vi "Paul_trap_scan.vi"() -> ()   [LabVIEW 2018]
uses:
  <instrlib>/AFG-2225/AFG-2225.lvlib
panel:
  in  "base name":string
  in  "Directory path":path=path "F:/data/20220803/3um_SiO2/1/pump/1"
  in  "stop 2 channels":bool
  in  "Single channel":bool
  in  "stop":bool
  in  "number of tests, Frequency":dbl
  in  "number of tests, Voltage":dbl
  in  "Frequency Step(kHz)":dbl=3.0 format="%.3g"
  in  "Voltage Step(V)":dbl=3.0 format="%.3g"
  in  "Delay Time 4+ (s)":dbl=1.0 caption="Delay Time (s)"
  in  "DC Offset (0.00 V)":dbl format="%.2g"
  in  "Frequency (kHz)":dbl=1000.0 format="%_7g"
  in  "Start Voltage (Vpp)":dbl=3.0 format="%.3g"
  in  "Waveform Function (0: Sine)":u16(ring) items=["Sine", "Square", "Pulse", "Ramp", "Noise"]
  in  "Impedance (0: 50 OHM)":u16(ring) items=["50 OHM", "High Z"]
  in  "Channel (0: CH1)":u16(ring) items=["CH1", "CH2"]
  # "Wait for a loop to end then stop"
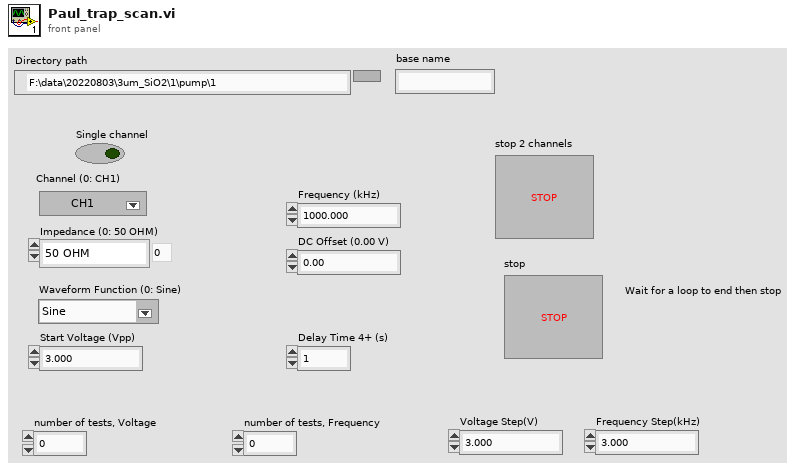
[diagram p1: front panel]
types:
  T1 = enum16{"open", "replace", "create", "open or create", "replace or create", "replace or create with confirmation"}
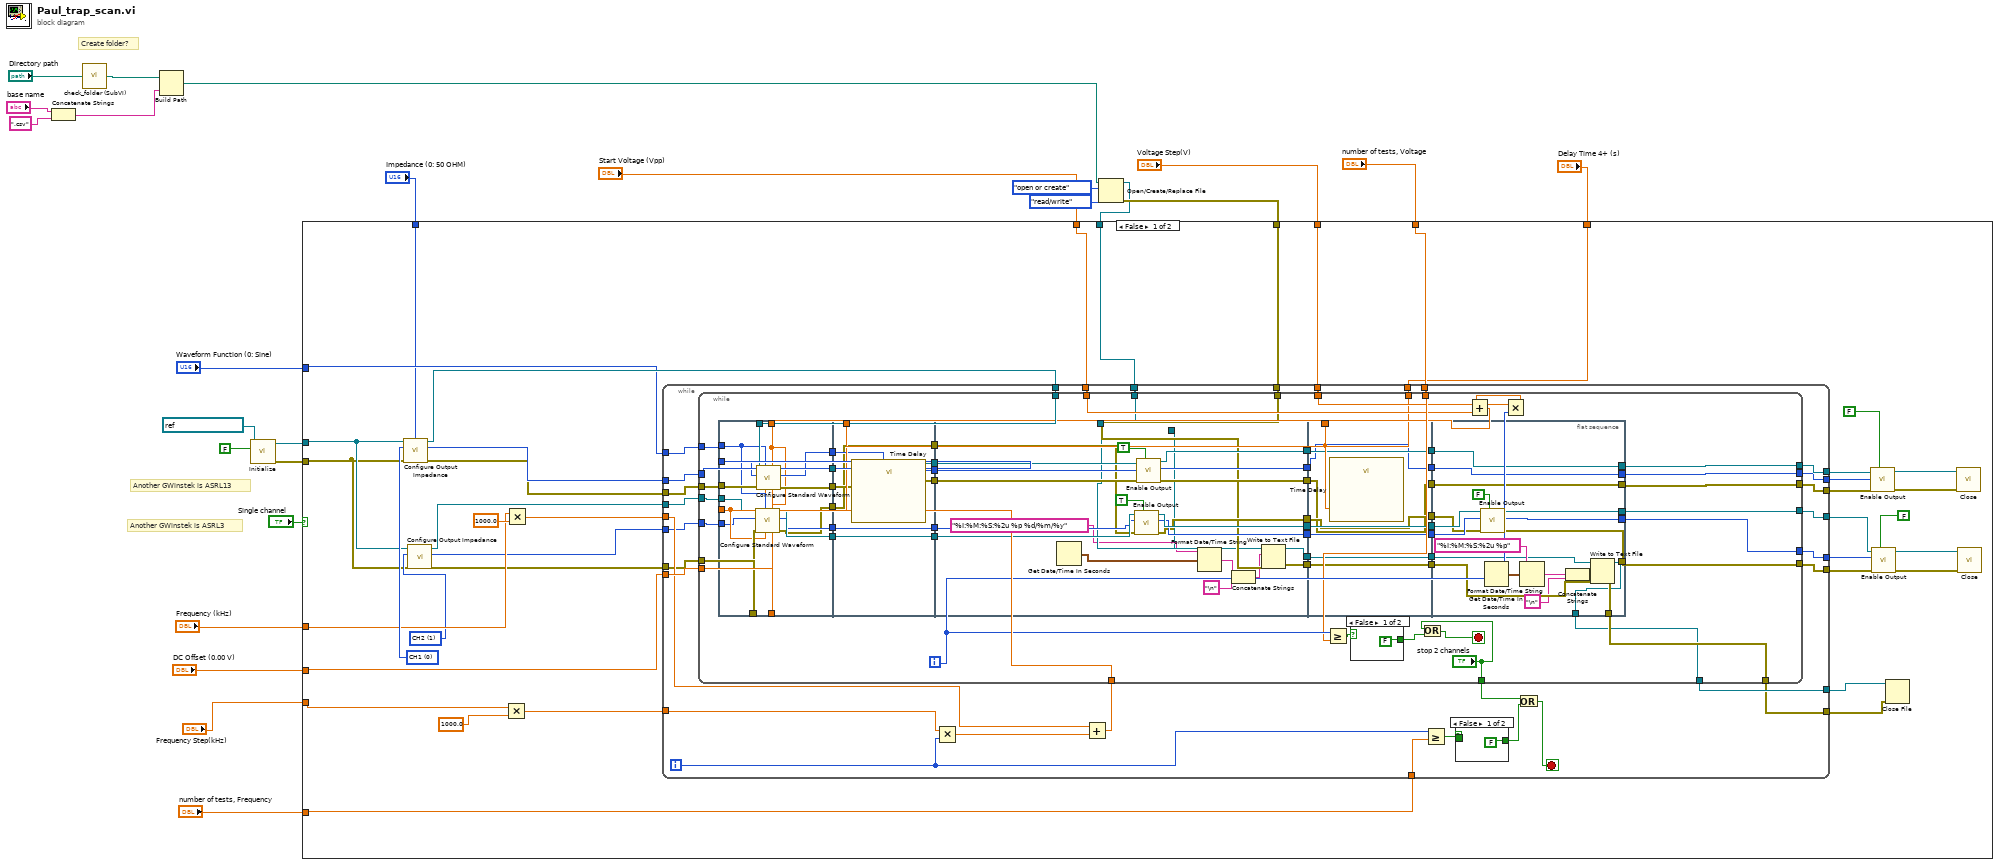
[diagram p0: block diagram]
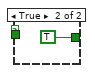
[diagram p2: hidden frame]
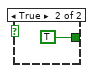
[diagram p3: hidden frame]
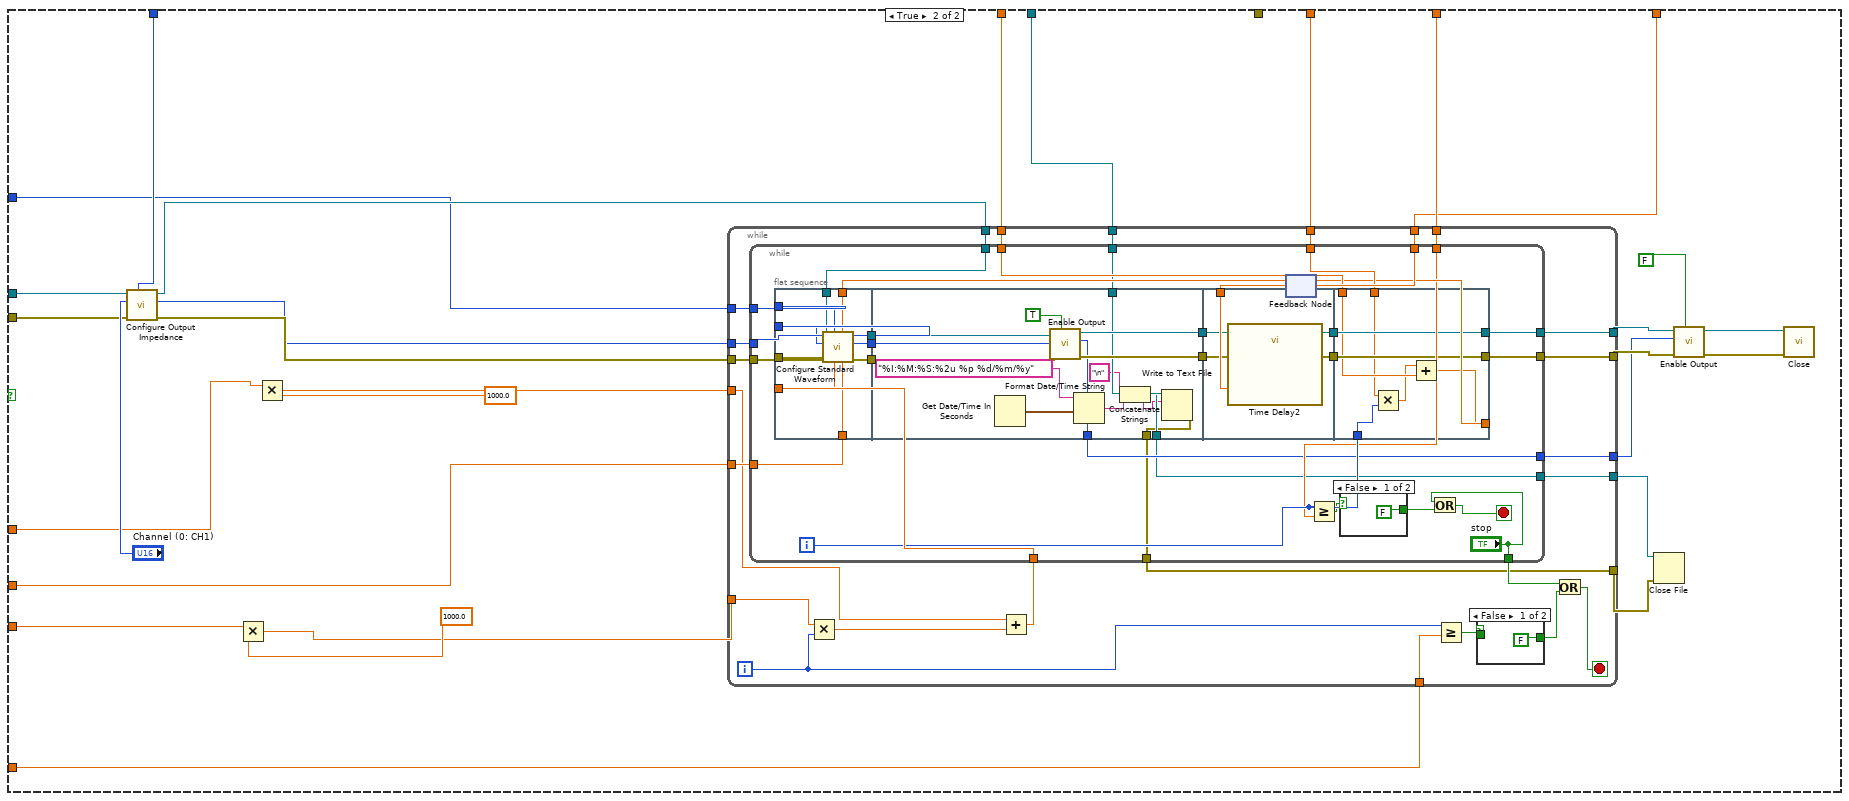
[diagram p4: hidden frame]
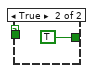
[diagram p5: hidden frame]
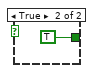
[diagram p6: hidden frame]
diagram:
  # "Create folder?"
  # "Another GWinstek is ASRL3"
  # "Another GWinstek is ASRL13"
  n1 = Concatenate Strings("base name", ".csv" ("string")) -> (w8:string)
  n2 = call "check_folder (SubVI).vi"("path in"="Directory path") -> ("path out"=w6:path)
  n3 = Build Path(base path=w6, name or relative path=w8) -> (appended path=w4:path)
  n4 = call <instrlib>:"Initialize.vi"("ID Query (True)"=FALSE, "VISA resource name"=refnum<visa-resource-name> "ASRL13::INSTR") -> ("error out"=w23:errorcluster, "VISA resource name out"=w24:refnum<visa-resource-name>)  [unwired: 8 in]
  n5 = Open/Create/Replace File(file path (use dialog)=w4, operation (0:open)=T1."open or create", access (0:read/write)=enum16{"read/write", "read-only", "write-only"}."read/write") -> (refnum out=w3:refnum<file>, error out=w5:errorcluster)  [unwired: 3 in, 1 out]
  n6 = case shown="False" "Single channel" {
    tunnel: w24 -> [w42 w261]
    tunnel: w23 -> [w41 w260]
    tunnel: "Impedance (0: 50 OHM)" -> [w30 w246]
    tunnel: "Start Voltage (Vpp)" -> [w52 w245]
    tunnel: "Voltage Step(V)" -> [w51 w244]
    tunnel: "number of tests, Voltage" -> [w50 w243]
    tunnel: "Delay Time 4+ (s)" -> [w49 w242]
    tunnel: "Waveform Function (0: Sine)" -> [w44 w241]
    tunnel: "Frequency (kHz)" -> [w45 w240]
    tunnel: "DC Offset (0.00 V)" -> [w46 w239]
    tunnel: "Frequency Step(kHz)" -> [w47 w238]
    tunnel: "number of tests, Frequency" -> [w48 w237]
    tunnel: w3 -> [w29 w236]
    tunnel: w5 -> [w28 _]
    frame False {
      w56 = u16 0 items=["CH1", "CH2"] ("Channel (0: CH1)")
      w43 = u16 1 items=["CH1", "CH2"] ("Channel (0: CH1)")
      n7 = call <instrlib>:"Configure Output Impedance.vi"("VISA resource name"=w42, "Channel (0: CH1)"=w56, "error in (no error)"=w41, "Impedance (0: 50 OHM)"=w30) -> ("VISA resource name out"=w59:refnum<visa-resource-name>, "Channel out"=w58:u16, "error out"=w57:errorcluster)  [unwired: 4 in]
      n8 = call <instrlib>:"Configure Output Impedance.vi"("VISA resource name"=w42, "Channel (0: CH1)"=w43, "error in (no error)"=w41) -> ("VISA resource name out"=w40:refnum<visa-resource-name>, "Channel out"=w31:u16, "error out"=w39:errorcluster)  [unwired: 5 in]
      n9 = Multiply(x=w47, y=1000.0) -> (x*y=w60:dbl)
      n10 = Multiply(x=w45, y=1000.0) -> (x*y=w61:dbl)
      n11 = while {
        tunnel: w49 -> [w97]
        tunnel: w46 -> [w96]
        tunnel: w52 -> [w95]
        tunnel: w61 -> [w86]
        tunnel: w44 -> [w94]
        tunnel: w57 -> [w93]
        tunnel: w58 -> [w92]
        tunnel: w59 -> [w91]
        tunnel: w51 -> [w90]
        tunnel: w50 -> [w89]
        tunnel: w60 -> [w88]
        tunnel: w48 -> [w81]
        tunnel: [w84] -> w63
        tunnel: [w83] -> w62
        tunnel: w40 -> [w76]
        tunnel: w39 -> [w75]
        tunnel: [w74] -> w35
        tunnel: [w73] -> w34
        tunnel: [w72] -> w33
        tunnel: [w71] -> w32
        tunnel: w31 -> [w70]
        tunnel: w29 -> [w69]
        tunnel: w28 -> [w68]
        tunnel: [w67] -> w27
        tunnel: [w66] -> w26
        i -> [w82]
        stop <- w78 stop-if-true
        n12 = Multiply(x=w88, y=w82) -> (x*y=w87:dbl)
        n13 = Add(x=w86, y=w87) -> (x+y=w85:dbl)
        n14 = while {
          tunnel: w97 -> [w137]
          tunnel: w96 -> [w157]
          tunnel: w95 -> [w143]
          tunnel: w94 -> [w156]
          tunnel: w93 -> [w155]
          tunnel: w92 -> [w154]
          tunnel: w91 -> [w153]
          tunnel: w90 -> [w142]
          tunnel: w89 -> [w148]
          tunnel: w85 -> [w152]
          tunnel: [w151] -> w84
          tunnel: [w150] -> w83
          tunnel: ["stop 2 channels"] -> w77
          tunnel: w76 -> [w139]
          tunnel: w75 -> [w138]
          tunnel: [w130] -> w74
          tunnel: [w129] -> w73
          tunnel: [w128] -> w72
          tunnel: [w123] -> w71
          tunnel: w70 -> [w120]
          tunnel: w69 -> [w118]
          tunnel: w68 -> [w119]
          tunnel: [w112] -> w67
          tunnel: [w113] -> w66
          i -> [w149]
          stop <- w145 stop-if-true
          n15 = flat-sequence {
            tunnel: [w171] -> w111
            tunnel: [w172] -> w109
            tunnel: [w173] -> w110
            tunnel: w157 -> [w165]
            tunnel: w140 -> [w167]
            tunnel: w152 -> [w166]
            tunnel: w156 -> [w168]
            tunnel: w155 -> [w175]
            tunnel: w154 -> [w160]
            tunnel: w153 -> [w174]
            tunnel: w139 -> [w170]
            tunnel: w138 -> [w169]
            tunnel: [w164] -> w108
            tunnel: [w163] -> w107
            tunnel: [w162] -> w106
            tunnel: w120 -> [w161]
            tunnel: w137 -> [w182]
            tunnel: w111 -> [w181]
            tunnel: w110 -> [w180]
            tunnel: [w180] -> w105
            tunnel: [w181] -> w104
            tunnel: [w179] -> w103
            tunnel: w109 -> [w179]
            tunnel: [w178] -> w102
            tunnel: w108 -> [w178]
            tunnel: [w177] -> w101
            tunnel: w107 -> [w177]
            tunnel: [w176] -> w100
            tunnel: w106 -> [w176]
            tunnel: w105 -> [w201]
            tunnel: w104 -> [w203]
            tunnel: w103 -> [w202]
            tunnel: w102 -> [w200]
            tunnel: w101 -> [w199]
            tunnel: w100 -> [w198]
            tunnel: [w197] -> w135
            tunnel: [w196] -> w133
            tunnel: [w195] -> w131
            tunnel: [w194] -> w126
            tunnel: [w193] -> w124
            tunnel: [w192] -> w121
            tunnel: w119 -> [w191]
            tunnel: w118 -> [w190]
            tunnel: [w187] -> _
            tunnel: [w187] -> w117
            tunnel: [w186] -> w115
            tunnel: w137 -> [w214]
            tunnel: [w213] -> w136
            tunnel: w135 -> [w213]
            tunnel: [w212] -> w134
            tunnel: w133 -> [w212]
            tunnel: [w211] -> w132
            tunnel: w131 -> [w211]
            tunnel: [w210] -> w127
            tunnel: w126 -> [w210]
            tunnel: [w209] -> w125
            tunnel: w124 -> [w209]
            tunnel: [w208] -> w122
            tunnel: w121 -> [w208]
            tunnel: w117 -> [w207]
            tunnel: [w207] -> w116
            tunnel: w115 -> [w206]
            tunnel: [w206] -> w114
            tunnel: [w226] -> w150
            tunnel: [w224] -> w151
            tunnel: w136 -> [w232]
            tunnel: w134 -> [w231]
            tunnel: w132 -> [w230]
            tunnel: [w229] -> w130
            tunnel: [w228] -> w129
            tunnel: [w227] -> w128
            tunnel: w127 -> [w226]
            tunnel: w125 -> [w225]
            tunnel: [w225] -> w123
            tunnel: w122 -> [w224]
            tunnel: w116 -> [w221]
            tunnel: w114 -> [w220]
            tunnel: [w219] -> w113
            tunnel: [w215] -> w112
            frame #0 {
              n16 = call <instrlib>:"Configure Standard Waveform.vi"("DC Offset (0.00 V)"=w165, "Amplitude (3.000 Vpp)"=w167, "Frequency (1000.000 Hz)"=w166, "Waveform Function (0: Sine)"=w168, "error in (no error)"=w169, "Channel (0: CH1)"=w161, "VISA resource name"=w170) -> ("error out"=w162:errorcluster, "Channel out"=w163:u16, "VISA resource name out"=w164:refnum<visa-resource-name>)  [unwired: 2 in]
              n17 = call <instrlib>:"Configure Standard Waveform.vi"("DC Offset (0.00 V)"=w165, "Amplitude (3.000 Vpp)"=w167, "Frequency (1000.000 Hz)"=w166, "Waveform Function (0: Sine)"=w168, "error in (no error)"=w175, "Channel (0: CH1)"=w160, "VISA resource name"=w174) -> ("error out"=w173:errorcluster, "Channel out"=w172:u16, "VISA resource name out"=w171:refnum<visa-resource-name>)  [unwired: 2 in]
            }
            frame #1 {
              n18 = call "Time Delay"("Delay Time (s)"=w182) -> ()  [unwired: 10 in, 1 out]
            }
            frame #2 {
              n19 = Get Date/Time In Seconds() -> (seconds since 1Jan1904=w189:timestamp)
              n20 = call <instrlib>:"Enable Output.vi"("Enable Output (T: Enable)"=TRUE, "error in (no error)"=w198, "Channel (0: CH1)"=w199, "VISA resource name"=w200) -> ("error out"=w195:errorcluster, "Channel out"=w196:u16, "VISA resource name out"=w197:refnum<visa-resource-name>)  [unwired: 5 in]
              n21 = call <instrlib>:"Enable Output.vi"("Enable Output (T: Enable)"=TRUE, "error in (no error)"=w201, "Channel (0: CH1)"=w202, "VISA resource name"=w203) -> ("error out"=w192:errorcluster, "Channel out"=w193:u16, "VISA resource name out"=w194:refnum<visa-resource-name>)  [unwired: 5 in]
              n22 = Format Date/Time String(time format string (%c)="%I:%M:%S:%2u %p %d/%m/%y", seconds (now)=w189) -> (date/time string=w184:string)  [unwired: 1 in]
              n23 = Concatenate Strings(w184, "\n" ("string")) -> (w185:string)
              n24 = Write to Text File(file (use dialog)=w190, text=w185, error in=w191) -> (refnum out=w187:refnum<file>, error out=w186:errorcluster)  [unwired: 1 in, 1 out]
            }
            frame #3 {
              n25 = call "Time Delay"("Delay Time (s)"=w214) -> ()  [unwired: 10 in, 1 out]
            }
            frame #4 {
              n26 = call <instrlib>:"Enable Output.vi"("Enable Output (T: Enable)"=FALSE, "error in (no error)"=w230, "Channel (0: CH1)"=w231, "VISA resource name"=w232) -> ("error out"=w227:errorcluster, "Channel out"=w228:u16, "VISA resource name out"=w229:refnum<visa-resource-name>)  [unwired: 5 in]
              n27 = Get Date/Time In Seconds() -> (seconds since 1Jan1904=w223:timestamp)
              n28 = Format Date/Time String(time format string (%c)="%I:%M:%S:%2u %p", seconds (now)=w223) -> (date/time string=w218:string)  [unwired: 1 in]
              n29 = Concatenate Strings(w218, "\n" ("string")) -> (w217:string)
              n30 = Write to Text File(file (use dialog)=w221, text=w217, error in=w220) -> (refnum out=w215:refnum<file>, error out=w219:errorcluster)  [unwired: 1 in, 1 out]
            }
          }
          n31 = Greater Or Equal?(x=w149, y=w148) -> (x >= y?=w147:bool)
          n32 = case shown="False" w147 {
            tunnel: [FALSE TRUE] -> w146
            frame False {
            }
            frame True {
            }
          }
          n33 = Or(x="stop 2 channels", y=w146) -> (x .or. y?=w145:bool)
          n34 = Multiply(x=w142, y=w149) -> (x*y=w141:dbl)
          n35 = Add(x=w141, y=w143) -> (x+y=w140:dbl)
        }
        n36 = Greater Or Equal?(x=w82, y=w81) -> (x >= y?=w80:bool)
        n37 = case shown="False" w80 {
          tunnel: [FALSE TRUE] -> w79
          tunnel: w80 -> [_ _]
          frame False {
          }
          frame True {
          }
        }
        n38 = Or(x=w77, y=w79) -> (x .or. y?=w78:bool)
      }
      n39 = call <instrlib>:"Enable Output.vi"("Enable Output (T: Enable)"=FALSE, "error in (no error)"=w63, "Channel (0: CH1)"=w32, "VISA resource name"=w62) -> ("error out"=w65:errorcluster, "VISA resource name out"=w64:refnum<visa-resource-name>)  [unwired: 5 in, 1 out]
      n40 = call <instrlib>:"Enable Output.vi"("Enable Output (T: Enable)"=FALSE, "error in (no error)"=w33, "Channel (0: CH1)"=w34, "VISA resource name"=w35) -> ("error out"=w38:errorcluster, "VISA resource name out"=w37:refnum<visa-resource-name>)  [unwired: 5 in, 1 out]
      n41 = Close File(refnum=w27, error in=w26) -> ()  [unwired: 2 out]
      n42 = call <instrlib>:"Close.vi"("error in (no error)"=w65, "VISA resource name"=w64) -> ()  [unwired: 9 in, 1 out]
      n43 = call <instrlib>:"Close.vi"("error in (no error)"=w38, "VISA resource name"=w37) -> ()  [unwired: 9 in, 1 out]
    }
    frame True {
      n44 = call <instrlib>:"Configure Output Impedance.vi"("VISA resource name"=w261, "Channel (0: CH1)"="Channel (0: CH1)", "error in (no error)"=w260, "Impedance (0: 50 OHM)"=w246) -> ("VISA resource name out"=w257:refnum<visa-resource-name>, "Channel out"=w258:u16, "error out"=w259:errorcluster)  [unwired: 4 in]
      n45 = Multiply(x=w238, y=1000.0) -> (x*y=w255:dbl)
      n46 = Multiply(x=w240, y=1000.0) -> (x*y=w254:dbl)
      n47 = while {
        tunnel: w242 -> [w287]
        tunnel: w239 -> [w286]
        tunnel: w245 -> [w285]
        tunnel: w254 -> [w276]
        tunnel: w241 -> [w284]
        tunnel: w259 -> [w283]
        tunnel: w258 -> [w282]
        tunnel: w257 -> [w281]
        tunnel: w244 -> [w280]
        tunnel: w243 -> [w279]
        tunnel: w255 -> [w278]
        tunnel: w237 -> [w271]
        tunnel: [w274] -> w250
        tunnel: [w273] -> w251
        tunnel: [w266] -> w247
        tunnel: w236 -> [w265]
        tunnel: [w264] -> w235
        tunnel: [w263] -> w234
        i -> [w272]
        stop <- w268 stop-if-true
        n48 = Multiply(x=w278, y=w272) -> (x*y=w277:dbl)
        n49 = Add(x=w276, y=w277) -> (x+y=w275:dbl)
        n50 = while {
          tunnel: w287 -> [w319]
          tunnel: w286 -> [w313]
          tunnel: w285 -> [w305]
          tunnel: w284 -> [w312]
          tunnel: w283 -> [w311]
          tunnel: w282 -> [w310]
          tunnel: w281 -> [w309]
          tunnel: w280 -> [w306]
          tunnel: w279 -> [w298]
          tunnel: w275 -> [w302]
          tunnel: [w301] -> w274
          tunnel: [w300] -> w273
          tunnel: ["stop"] -> w267
          tunnel: [w293] -> w266
          tunnel: w265 -> [w292]
          tunnel: [w291] -> w264
          tunnel: [w290] -> w263
          i -> [w299]
          stop <- w295 stop-if-true
          n51 = flat-sequence {
            tunnel: [w323] -> w316
            tunnel: [w324] -> w315
            tunnel: [w325] -> w314
            tunnel: w313 -> [w331]
            tunnel: w303 -> [w322]
            tunnel: w302 -> [w330]
            tunnel: w312 -> [w329]
            tunnel: w311 -> [w328]
            tunnel: w310 -> [w327]
            tunnel: w309 -> [w326]
            tunnel: [w342] -> w318
            tunnel: [w341] -> w317
            tunnel: w316 -> [w346]
            tunnel: w315 -> [w345]
            tunnel: w314 -> [w344]
            tunnel: [w340] -> w293
            tunnel: w292 -> [w337]
            tunnel: [w336] -> w291
            tunnel: [w335] -> w290
            tunnel: w319 -> [w349]
            tunnel: w318 -> [w348]
            tunnel: w317 -> [w347]
            tunnel: [w347] -> w308
            tunnel: [w348] -> w307
            tunnel: [w355] -> w300
            tunnel: [w356] -> w301
            tunnel: w308 -> [w356]
            tunnel: w307 -> [w355]
            tunnel: w306 -> [w351]
            tunnel: w305 -> [w354]
            tunnel: w299 -> [w353]
            tunnel: [w350] -> w304
            frame #0 {
              n52 = call <instrlib>:"Configure Standard Waveform.vi"("DC Offset (0.00 V)"=w331, "Amplitude (3.000 Vpp)"=w322, "Frequency (1000.000 Hz)"=w330, "Waveform Function (0: Sine)"=w329, "error in (no error)"=w328, "Channel (0: CH1)"=w327, "VISA resource name"=w326) -> ("error out"=w325:errorcluster, "Channel out"=w324:u16, "VISA resource name out"=w323:refnum<visa-resource-name>)  [unwired: 2 in]
            }
            frame #1 {
              n53 = Get Date/Time In Seconds() -> (seconds since 1Jan1904=w338:timestamp)
              n54 = call <instrlib>:"Enable Output.vi"("Enable Output (T: Enable)"=TRUE, "error in (no error)"=w344, "Channel (0: CH1)"=w345, "VISA resource name"=w346) -> ("error out"=w341:errorcluster, "Channel out"=w340:u16, "VISA resource name out"=w342:refnum<visa-resource-name>)  [unwired: 5 in]
              n55 = Format Date/Time String(time format string (%c)="%I:%M:%S:%2u %p %d/%m/%y", seconds (now)=w338) -> (date/time string=w334:string)  [unwired: 1 in]
              n56 = Concatenate Strings(w334, "\n" ("string")) -> (w332:string)
              n57 = Write to Text File(file (use dialog)=w337, text=w332) -> (refnum out=w336:refnum<file>, error out=w335:errorcluster)  [unwired: 2 in, 1 out]
            }
            frame #2 {
              n58 = call "Time Delay2"("Delay Time (s)"=w349) -> ()  [unwired: 10 in, 1 out]
            }
            frame #3 {
              n59 = Multiply(x=w351, y=w353) -> (x*y=w352:dbl)
              n60 = Add(x=w352, y=w354) -> (x+y=w350:dbl)
            }
          }
          n61 = feedback-in #1(w304) -> ()
          n62 = feedback #1() -> (w303:dbl)  [unwired: 1 in]
          n63 = Greater Or Equal?(x=w299, y=w298) -> (x >= y?=w297:bool)
          n64 = case shown="False" w297 {
            tunnel: [FALSE TRUE] -> w296
            frame False {
            }
            frame True {
            }
          }
          n65 = Or(x="stop", y=w296) -> (x .or. y?=w295:bool)
        }
        n66 = Greater Or Equal?(x=w272, y=w271) -> (x >= y?=w270:bool)
        n67 = case shown="False" w270 {
          tunnel: [FALSE TRUE] -> w269
          tunnel: w270 -> [_ _]
          frame False {
          }
          frame True {
          }
        }
        n68 = Or(x=w267, y=w269) -> (x .or. y?=w268:bool)
      }
      n69 = Close File(refnum=w235, error in=w234) -> ()  [unwired: 2 out]
      n70 = call <instrlib>:"Enable Output.vi"("Enable Output (T: Enable)"=FALSE, "error in (no error)"=w250, "Channel (0: CH1)"=w247, "VISA resource name"=w251) -> ("error out"=w248:errorcluster, "VISA resource name out"=w249:refnum<visa-resource-name>)  [unwired: 5 in, 1 out]
      n71 = call <instrlib>:"Close.vi"("error in (no error)"=w248, "VISA resource name"=w249) -> ()  [unwired: 9 in, 1 out]
    }
  }
